vi "Get Connection ID.vi"(8 "Error In":errorcluster, 11 "TCP Network Connection in":refnum<k5>) -> (0 "Error Out":errorcluster, 3 "ConnectionID":string)   [LabVIEW 2014, in "hse-db.lvlib" / "MySQL (TCP).lvlib"]
uses:
  MySQL (TCP).lvlib
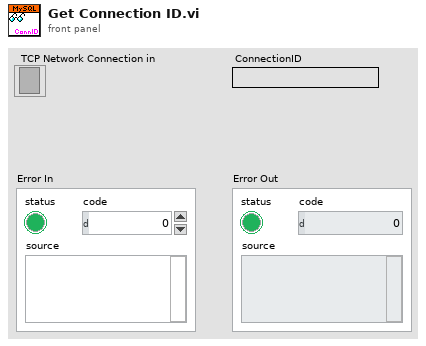
[diagram p1: front panel]
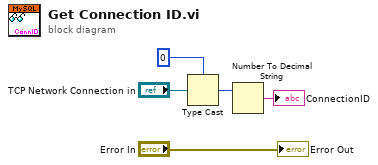
[diagram p0: block diagram]
diagram:
  n1 = Type Cast(type=u32 0, x="TCP Network Connection in") -> (*(type *) &x=w3:u32)
  n2 = Number To Decimal String(number=w3) -> (decimal integer string=→"ConnectionID":string)  [unwired: 1 in]
  "Error Out" <- "Error In"
